vi "Poisson Random.vi"(6 "seed":i32=-1, 7 "reset":bool, 10 "lambda":dbl=1.0, 11 "samples":i32=128) -> (0 "error":i32, 3 "Poisson random data":i32[](array[numeric]))   [LabVIEW 2010, in "NI_Gmath.lvlib"]
doc: "Generates random values from a variate X, where X describes the selected distribution type. You must manually select the polymorphic instance to use."
uses:
  NI_Gmath.lvlib
  st_error_code.ctl
panel:
  # "Poisson Random"
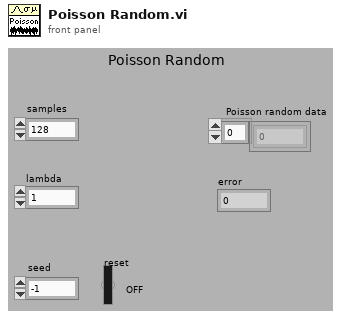
[diagram p1: front panel]
types:
  T1 = typedef "NI_Gmath.lvlib/st_error_code.ctl" = i32
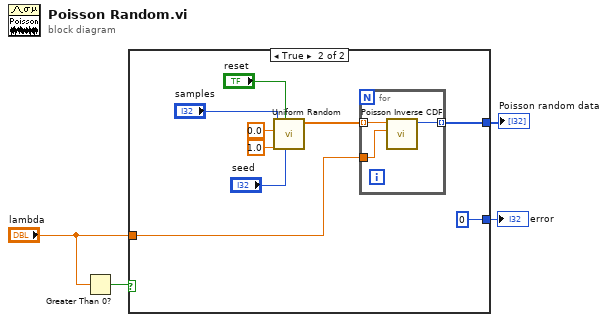
[diagram p0: block diagram]
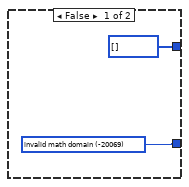
[diagram p2: hidden frame]
diagram:
  n1 = Greater Than 0?(x="lambda") -> (x > 0?=w2:bool)
  n2 = case shown="True" w2 {
    tunnel: [i32[] [] w9] -> w4
    tunnel: "lambda" -> [_ w8]
    tunnel: [w5 0 ("invalid math domain")] -> w1
    frame False {
      w5 = T1 -20069 items=["invalid math domain"=-20069, "Fourier interpolation size m >= n"=-20070, "empty array"=-20003] ("stat interp error code")
    }
    frame True {
      n3 = call "Uniform Random.vi"("seed"="seed", "reset"="reset", "xmax"=1.0, "xmin"=0.0, "samples"="samples") -> ("uniform random data"=w12:dbl[])  [unwired: 5 in, 1 out]
      n4 = for {
        tunnel: w12 -> [w17] mode=indexing
        tunnel: w8 -> [w18]
        tunnel: [w16] -> w9 mode=indexing
        n5 = call "Poisson Inverse CDF.vi"("lambda"=w18, "cdf(x)"=w17) -> ("x"=w16:i32)  [unwired: 8 in, 1 out]
      }
    }
  }
  "error" <- w1
  "Poisson random data" <- w4
